vi "Register.vi"(6 "Start Imidiatlely?(T)":bool=TRUE, 8 "error in (no error)":errorcluster, 10 "TimePeroid(ms)":i32, 11 "Name":string) -> (0 "error out":errorcluster, 3 "TimeupEvent":T1)   [LabVIEW 2017, in "TimerEngine.lvlib" / "TimerEngine.lvclass"]
uses:
  TimerEngine.lvclass
  _Typedef/Timer-UserEvent.ctl
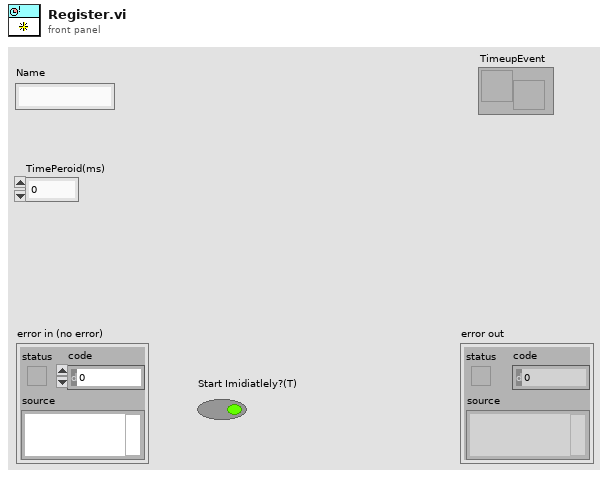
[diagram p1: front panel]
types:
  T1 = typedef "TimerEngine.lvlib/TimerEngine.lvclass/Timer-Userevent.ctl" = refnum<user-event>
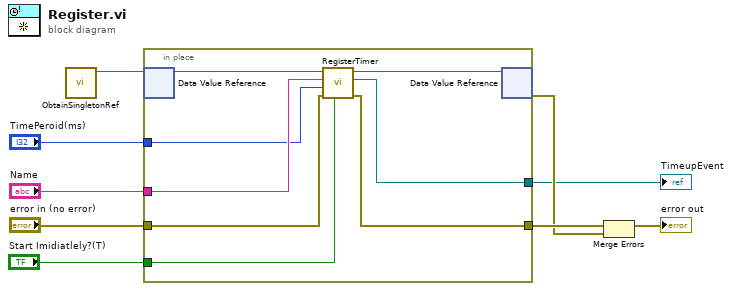
[diagram p0: block diagram]
diagram:
  n1 = call "ObtainSingletonRef.vi"() -> ("data value reference"=w9:refnum<data-value>)  [unwired: 10 in, 1 out]
  n2 = in-place {
    in-place-border: [w14] -> w8
    in-place-border: "error in (no error)" -> [w15]
    in-place-border: "Name" -> [w13]
    in-place-border: "TimePeroid(ms)" -> [w12]
    in-place-border: [w11] -> w2
    in-place-border: "Start Imidiatlely?(T)" -> [w10]
    n3 = in-place-dvr #1(w9) -> (w17:refnum<class "TimerEngine.lvclass">)  [unwired: 1 out]
    n4 = call "RegisterTimer.vi"("Start Imidiatlely?(F)"=w10, "error in (no error)"=w15, "TimePeroid(ms)"=w12, "Name"=w13, "UserEventTimer in"=w17) -> ("error out"=w14:errorcluster, "UserEvent"=w11:T1, "UserEventTimer out"=w16:refnum<class "TimerEngine.lvclass">)  [unwired: 4 in]
    n5 = in-place-dvr #1(w16) -> (w5:errorcluster)  [unwired: 1 out]
  }
  "TimeupEvent" <- w2
  n6 = Merge Errors(w8, w5) -> (→"error out":errorcluster)
